vi "Polymorphic test.vi"   [LabVIEW 2009]
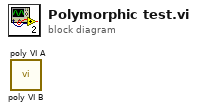
[diagram p0: block diagram]
diagram:
  n1 = call "poly VI B.vi"() -> ()  [unwired: 1 in]
  n2 = call "poly VI A.vi"() -> ()  [unwired: 1 in]
